vi "Log Text.vi"(8 "Error In":errorcluster, 10 "text":string, 11 "Log File Ref In":refnum<file>) -> (0 "Error Out":errorcluster, 3 "Log File Ref Out":refnum<file>)   [LabVIEW 2018]
doc: "Author: Scott Hannahs <sth@magnet.fsu.edu>\nCopyright 2018 Florida State University, All rights reserved."
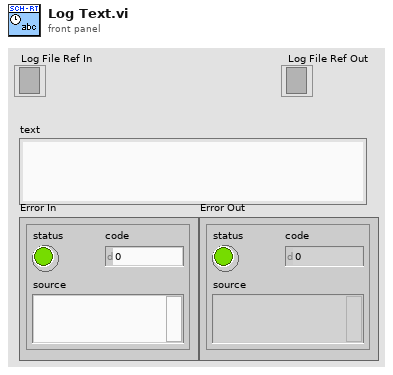
[diagram p1: front panel]
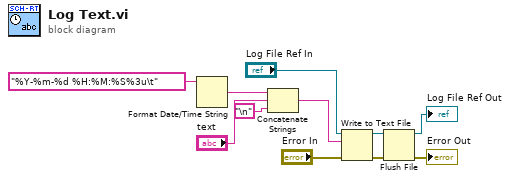
[diagram p0: block diagram]
diagram:
  n1 = Format Date/Time String(time format string (%c)="%Y-%m-%d %H:%M:%S%3u\t") -> (date/time string=w4:string)  [unwired: 2 in]
  n2 = Concatenate Strings(w4, "text", "\n") -> (w6:string)
  n3 = Write to Text File(file (use dialog)="Log File Ref In", text=w6, error in="Error In") -> (refnum out=w7:refnum<file>, error out=w9:errorcluster)  [unwired: 1 in, 1 out]
  n4 = Flush File(refnum=w7, error in=w9) -> (refnum out=→"Log File Ref Out":refnum<file>, error out=→"Error Out":errorcluster)
